vi "Read -- Write Shell Test.vi"() -> ()   [LabVIEW 2014]
panel:
  in  "Waveform index for Write":i32
  out "WaveformData Write":T1
  out "Waveform Graph Write":waveform(dbl)(graph)
  out "Waveform Graph":waveform(dbl)(graph)
  out "WaveformData":T1
  in  "stop":bool
  in  "Waveform index":i32
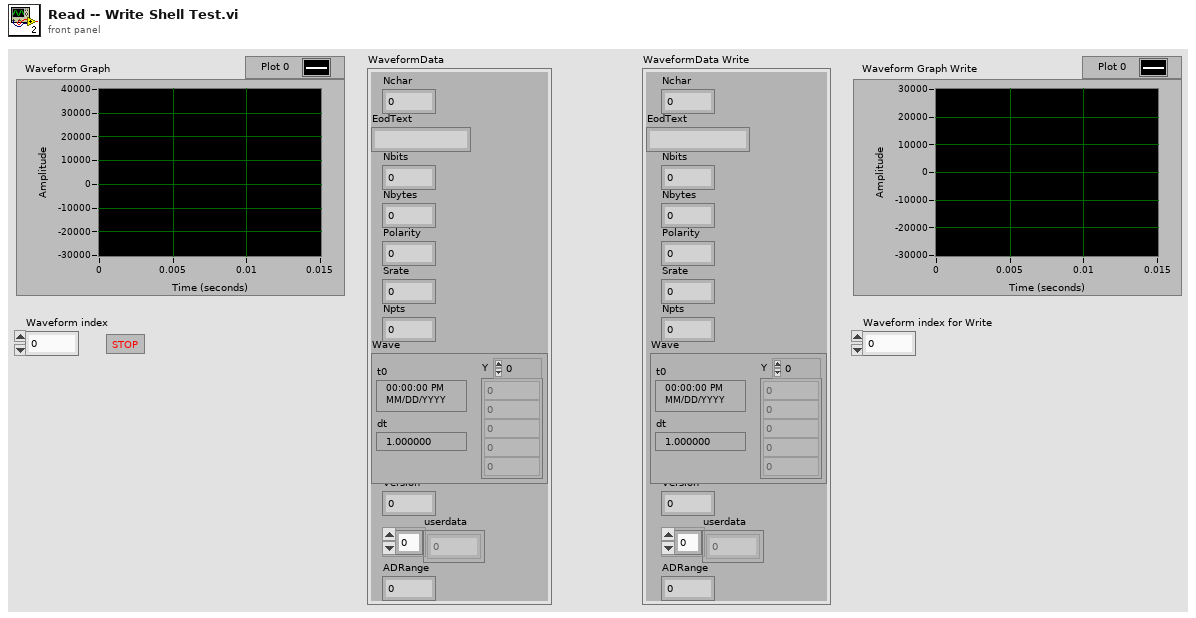
[diagram p1: front panel]
types:
  T1 = cluster{"Nchar":i32, "EodText":string, "Nbits":i32, "Nbytes":i32, "Polarity":i32, "Srate":i32, "Npts":i32, "Wave":waveform(dbl), "Version":i32, "userdata":dbl[], "ADRange":dbl}
  T2 = cluster{"Nchar":i32, "EodText":string, "Nbits":i32, "Nbytes":i32, "Polarity":i32, "Srate":i32, "Npts":i32, "Wave":waveform(dbl), "Version":i32, "userdata":dbl[], "ADRange":dbl}[]
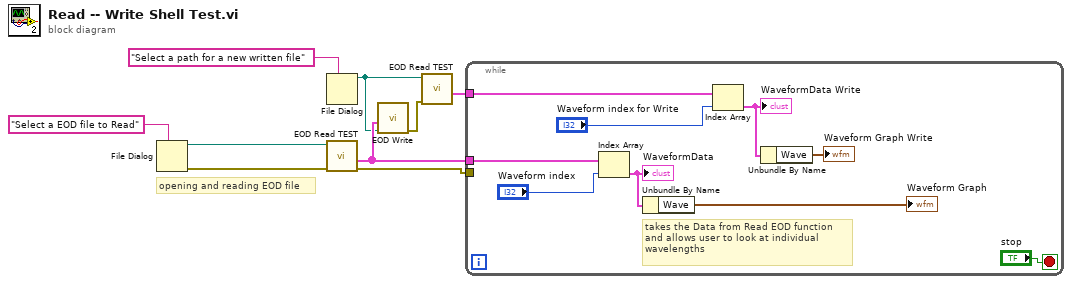
[diagram p0: block diagram]
diagram:
  # "opening and reading EOD file"
  n1 = File Dialog(7:"Select a EOD file to Read" ("prompt")) -> (0:w5:errorcluster, 3:w6:path)  [unwired: 6 in, 2 out]
  n2 = File Dialog(7:"Select a path for a new written file" ("prompt")) -> (3:w1:path)  [unwired: 6 in, 3 out]
  n3 = call "EOD Read TEST.vi"("error in (no error)"=w5, "Path"=w6) -> ("error out"=w4:errorcluster, "EODDataOut"=w3:T2)  [unwired: 7 in, 1 out]
  n4 = call "EOD Write.vi"("file path (use dialog)"=w1, "EODDataInput"=w3) -> ("error out"=w2:errorcluster)  [unwired: 7 in, 2 out]
  n5 = call "EOD Read TEST.vi"("error in (no error)"=w2, "Path"=w1) -> ("EODDataOut"=w9:T2)  [unwired: 7 in, 2 out]
  n6 = while {
    tunnel: w3 -> [w14]
    tunnel: w4 -> [_]
    tunnel: w9 -> [w10]
    stop <- "stop" stop-if-true
    # "takes the Data from Read EOD function\nand allows user to look at individual\nwavelengths"
    n7 = Index Array(array=w14, index="Waveform index") -> (element=w15:T1)
    "WaveformData" <- w15
    n8 = Unbundle By Name(w15) -> ("Wave"=→"Waveform Graph":waveform(dbl))
    n9 = Index Array(array=w10, index="Waveform index for Write") -> (element=w11:T1)
    "WaveformData Write" <- w11
    n10 = Unbundle By Name(w11) -> ("Wave"=→"Waveform Graph Write":waveform(dbl))
  }
